vi "Initialize.vi"(8 "error in (no error)":errorcluster, 11 "Network Device in":refnum<class "Network Device.lvclass">=refnum) -> (0 "error out":errorcluster, 3 "Network Device out":refnum<class "Network Device.lvclass">)   [LabVIEW 2019, in "Network Device.lvclass"]
uses:
  Network Device.lvclass
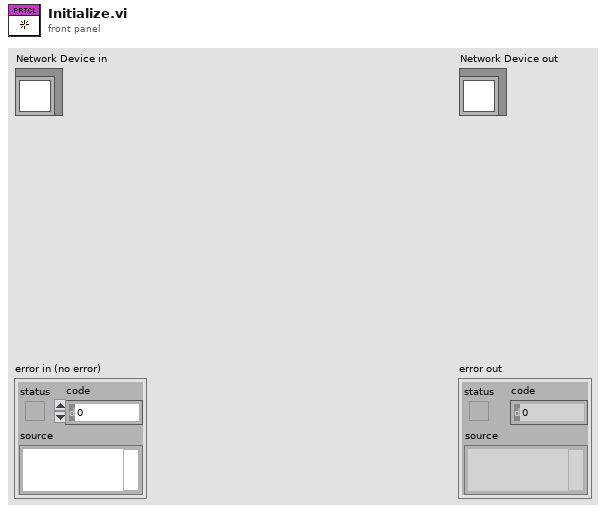
[diagram p1: front panel]
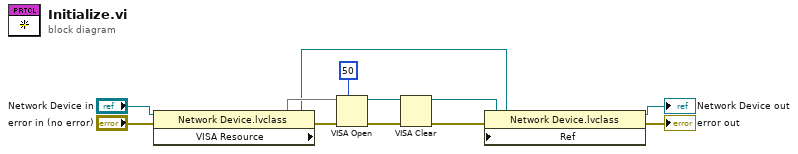
[diagram p0: block diagram]
diagram:
  n1 = property class="Network Device.lvclass"(reference="Network Device in", error in="error in (no error)") -> (reference out=w9:refnum<class "Network Device.lvclass">, error out=w10:errorcluster, "VISA Resource"=w12)
  n2 = VISA Open(timeout (0)=u32 50 ("VISA Open timeout (0)"), error in (no error)=w10, VISA resource name=w12) -> (VISA resource name=w8:refnum<visa-resource-name>, error out=w6:errorcluster)  [unwired: 2 in]
  n3 = VISA Clear(VISA resource name=w8, error in (no error)=w6) -> (VISA resource name out=w7:refnum<visa-resource-name>, error out=w5:errorcluster)
  n4 = property class="Network Device.lvclass"(reference=w9, error in=w5, "Ref"=w7) -> (reference out=→"Network Device out":refnum<class "Network Device.lvclass">, error out=→"error out":errorcluster)
